vi "Test.vi"   [LabVIEW 2014]
doc: "This VI is called when test mode begins, and will automatically be terminated when it ends. You can add manual or automatic tests and invoke them from the dashboard."
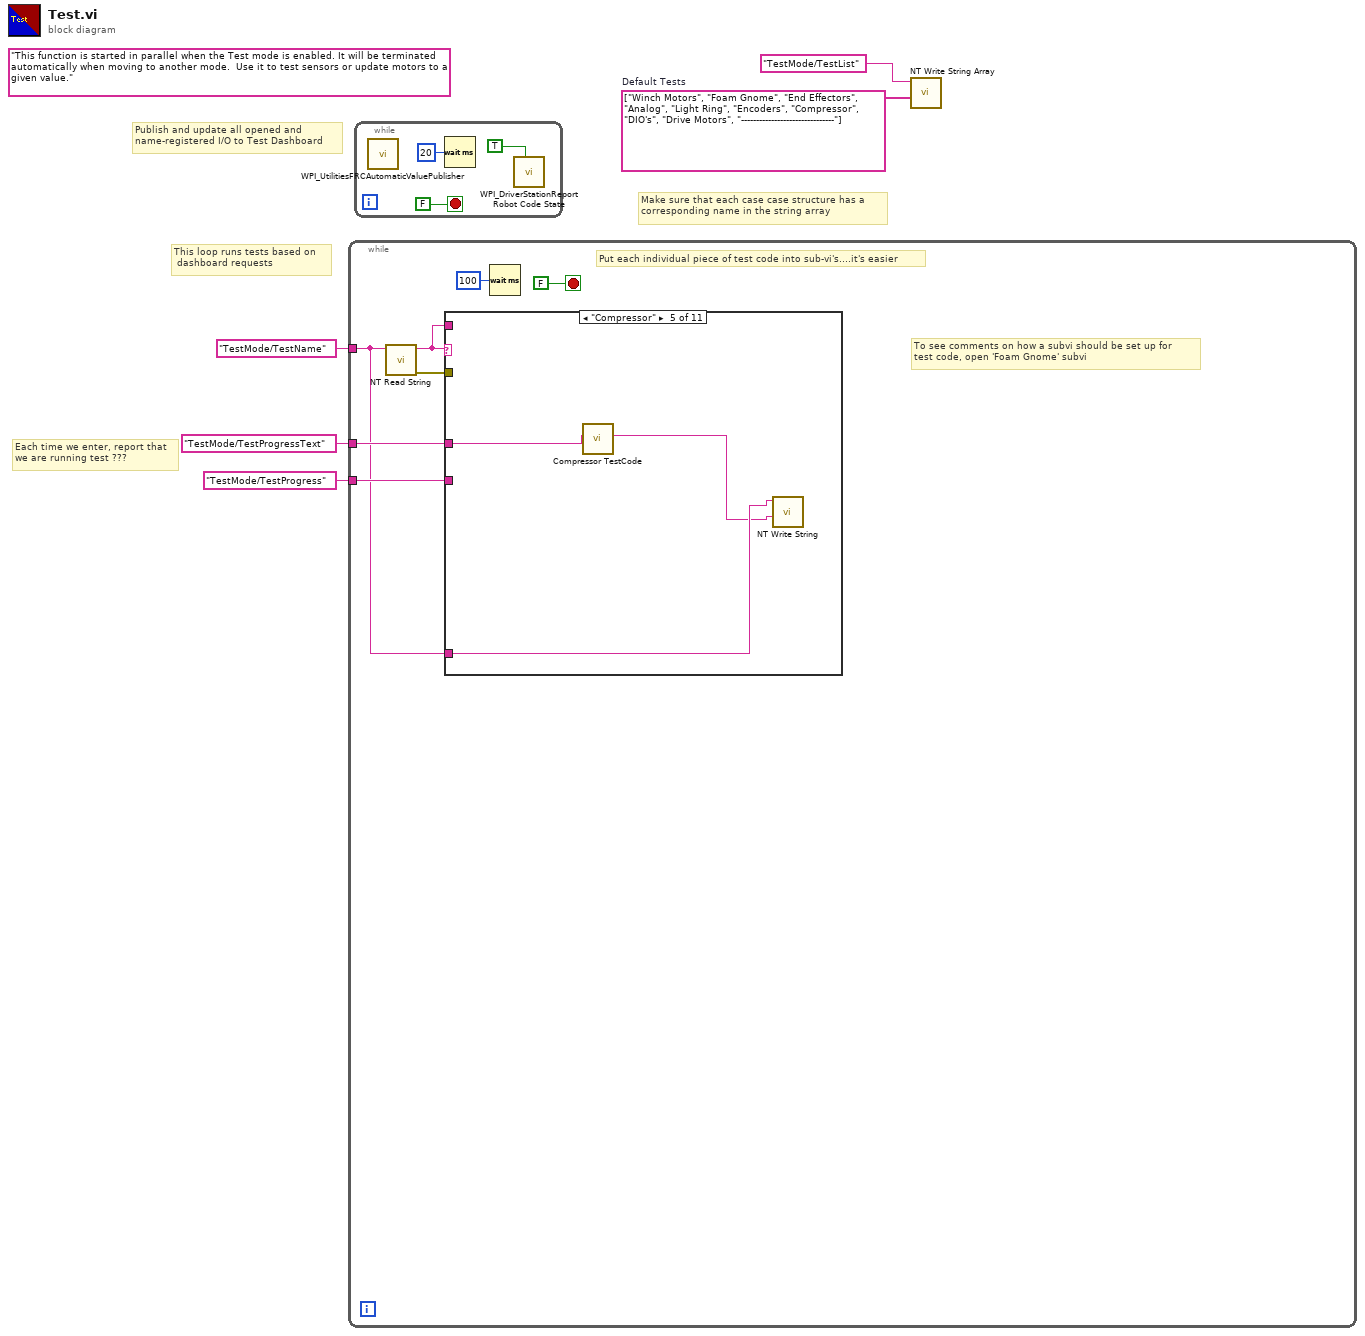
[diagram p0: block diagram]
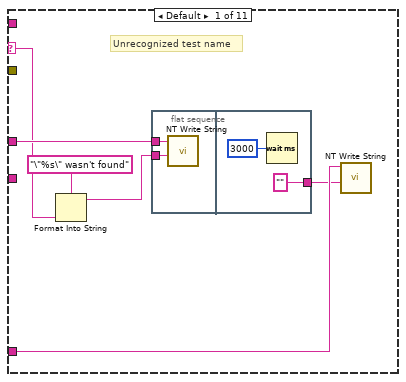
[diagram p2: hidden frame]
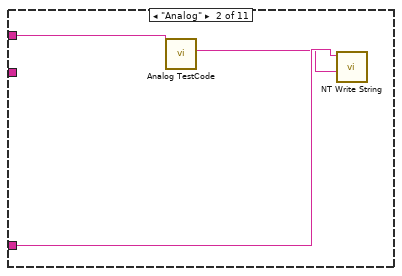
[diagram p3: hidden frame]
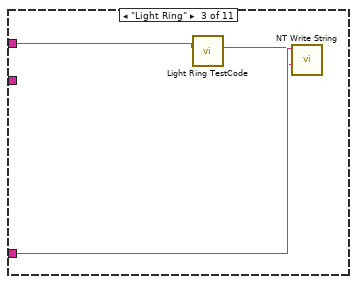
[diagram p4: hidden frame]
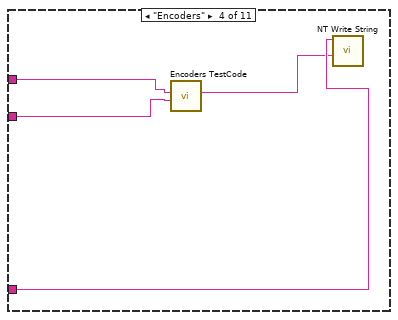
[diagram p5: hidden frame]
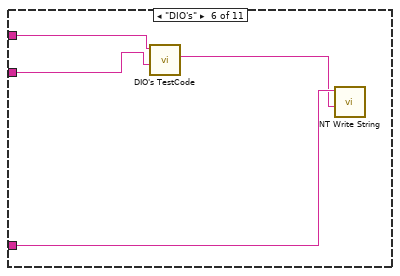
[diagram p6: hidden frame]
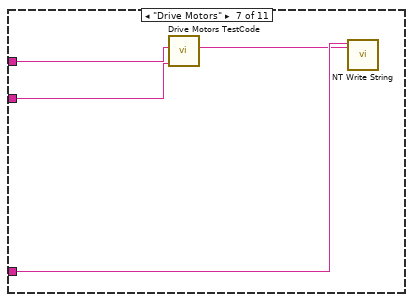
[diagram p7: hidden frame]
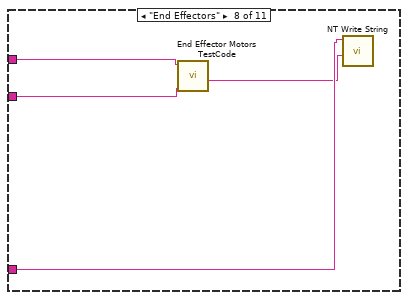
[diagram p8: hidden frame]
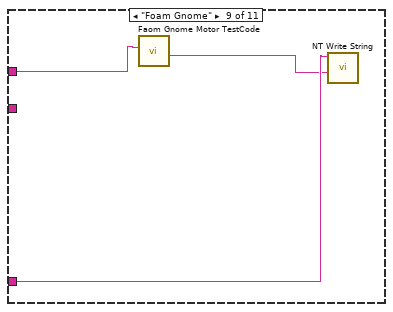
[diagram p9: hidden frame]
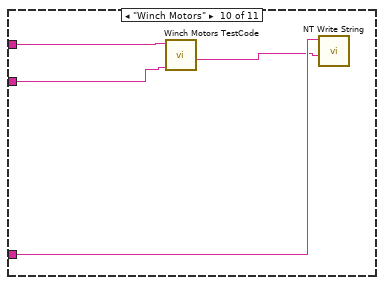
[diagram p10: hidden frame]
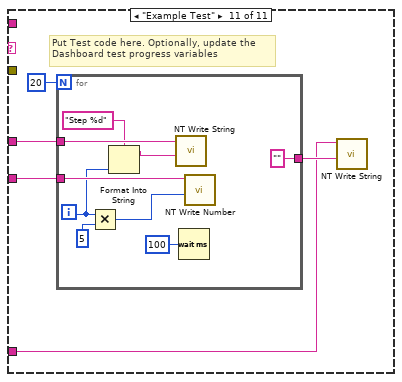
[diagram p11: hidden frame]
diagram:
  w2 = string[] ["Winch Motors", "Foam Gnome", "End Effectors", "Analog", "Light Ring", "Encoders", "Compressor", "DIO's", "Drive Motors", "-------------------------------"]  # Default Tests
  (unwired) "This function is started in parallel when the Test mode is enabled. It will be terminated automatically when moving to another mode.  Use it to test sensors or update motors to a given value."
  # "Make sure that each case case structure has a \ncorresponding name in the string array"
  # "This loop runs tests based on \n dashboard requests"
  # "Publish and update all opened and\nname-registered I/O to Test Dashboard"
  # "Each time we enter, report that\nwe are running test ???"
  n1 = while {
    tunnel: "TestMode/TestName" ("Name") -> [w7]
    tunnel: "TestMode/TestProgressText" ("Name") -> [w10]
    tunnel: "TestMode/TestProgress" ("Name") -> [w9]
    stop <- FALSE stop-if-true
    # "To see comments on how a subvi should be set up for\ntest code, open 'Foam Gnome' subvi"
    # "Put each individual piece of test code into sub-vi's....it's easier"
    n2 = call <vilib>:"NT Read String.vi"("Name"=w7) -> ("error out"=w6:errorcluster, "String"=w8:string)  [unwired: 9 in]
    n3 = case shown="\"Compressor\"" w8 {
      selector: w8 -> [w17 _ _ _ _ _ _ _ _ _ _]
      tunnel: w7 -> [w14 w25 w27 w32 w35 w39 w43 w47 w50 w54 w55]
      tunnel: w10 -> [w18 w23 w28 w31 w34 w38 w42 w46 w49 w52 w58]
      tunnel: w9 -> [_ _ _ w30 _ w37 w41 w45 _ w51 w59]
      tunnel: w8 -> [_ _ _ _ _ _ _ _ _ _ _]
      tunnel: w6 -> [_ _ _ _ _ _ _ _ _ _ _]
      frame Default {
        # "Unrecognized test name"
        n4 = Format Into String(format string="\"%s\" wasn't found" ("Name"), w17) -> (resulting string=w16:string)  [unwired: 2 in, 1 out]
        n5 = flat-sequence {
          tunnel: w18 -> [w19]
          tunnel: w16 -> [w20]
          tunnel: ["" ("Name")] -> w13
          frame #0 {
            n6 = call <vilib>:"NT Write String.vi"("String"=w20, "Name"=w19) -> ()  [unwired: 9 in, 1 out]
          }
          frame #1 {
            n7 = Wait (ms)(milliseconds to wait=u32 3000) -> ()  [unwired: 1 out]
          }
        }
        n8 = call <vilib>:"NT Write String.vi"("String"=w13, "Name"=w14) -> ()  [unwired: 9 in, 1 out]
      }
      frame "Analog" {
        n9 = call "Analog TestCode.vi"(10:w23) -> ("String"=w24:string)  [unwired: 10 in]
        n10 = call <vilib>:"NT Write String.vi"("String"=w24, "Name"=w25) -> ()  [unwired: 9 in, 1 out]
      }
      frame "Light Ring" {
        n11 = call "Light Ring TestCode.vi"("Step Text"=w28) -> ("Light Ring Output"=w26:string)  [unwired: 10 in]
        n12 = call <vilib>:"NT Write String.vi"("String"=w26, "Name"=w27) -> ()  [unwired: 9 in, 1 out]
      }
      frame "Encoders" {
        n13 = call "Encoders TestCode.vi"(1:"Step Text"=w31, 2:"Step Text"=w30) -> ("Encoders Output"=w29:string)  [unwired: 8 in]
        n14 = call <vilib>:"NT Write String.vi"("String"=w29, "Name"=w32) -> ()  [unwired: 9 in, 1 out]
      }
      frame "Compressor" {
        n15 = call "Compressor TestCode.vi"("Step Text"=w34) -> ("Compressor Output"=w33:string)  [unwired: 10 in]
        n16 = call <vilib>:"NT Write String.vi"("String"=w33, "Name"=w35) -> ()  [unwired: 9 in, 1 out]
      }
      frame "DIO's" {
        n17 = call "DIO's TestCode.vi"(9:"Step Text"=w37, 11:"Step Text"=w38) -> ("DIO Output"=w36:string)  [unwired: 9 in]
        n18 = call <vilib>:"NT Write String.vi"("String"=w36, "Name"=w39) -> ()  [unwired: 9 in, 1 out]
      }
      frame "Drive Motors" {
        n19 = call "Drive Motors TestCode.vi"(8:"Step Text"=w41, 10:"Step Text"=w42) -> ("Drive Motors Output"=w40:string)  [unwired: 9 in]
        n20 = call <vilib>:"NT Write String.vi"("String"=w40, "Name"=w43) -> ()  [unwired: 9 in, 1 out]
      }
      frame "End Effectors" {
        n21 = call "End Effector Motors TestCode.vi"(0:"Step Text"=w46, 3:"Step Text"=w45) -> ("Drive Motors Output"=w44:string)  [unwired: 7 in]
        n22 = call <vilib>:"NT Write String.vi"("String"=w44, "Name"=w47) -> ()  [unwired: 9 in, 1 out]
      }
      frame "Foam Gnome" {
        n23 = call "Faom Gnome Motor TestCode.vi"("Step Text"=w49) -> ("Foam Gnome Output"=w48:string)  [unwired: 10 in]
        n24 = call <vilib>:"NT Write String.vi"("String"=w48, "Name"=w50) -> ()  [unwired: 9 in, 1 out]
      }
      frame "Winch Motors" {
        n25 = call "Winch Motors TestCode.vi"(8:"Step Text"=w51, 11:"Step Text"=w52) -> ("Winch Motors Output"=w53:string)  [unwired: 9 in]
        n26 = call <vilib>:"NT Write String.vi"("String"=w53, "Name"=w54) -> ()  [unwired: 9 in, 1 out]
      }
      frame "Example Test" {
        # "Put Test code here. Optionally, update the\nDashboard test progress variables"
        n27 = for {
          N: 20 -> [_]
          tunnel: w59 -> [w68]
          tunnel: w58 -> [w66]
          tunnel: ["" ("String")] -> w56
          i -> [w63]
          n28 = Multiply(x=w63, y=u32 5 ("milliseconds to wait")) -> (x*y=w64:u32)
          n29 = Format Into String(format string="Step %d", w63) -> (resulting string=w61:string)  [unwired: 2 in, 1 out]
          n30 = call <vilib>:"NT Write String.vi"("String"=w61, "Name"=w66) -> ()  [unwired: 9 in, 1 out]
          n31 = Wait (ms)(milliseconds to wait=u32 100) -> ()  [unwired: 1 out]
          n32 = call <vilib>:"NT Write Number.vi"("Numeric"=w64, "Name"=w68) -> ()  [unwired: 9 in, 1 out]
        }
        n33 = call <vilib>:"NT Write String.vi"("String"=w56, "Name"=w55) -> ()  [unwired: 9 in, 1 out]
      }
    }
    n34 = Wait (ms)(milliseconds to wait=u32 100) -> ()  [unwired: 1 out]
  }
  n35 = while {
    stop <- FALSE stop-if-true
    n36 = call <vilib>:"WPI_UtilitiesFRCAutomaticValuePublisher.vi"() -> ()  [unwired: 12 in]
    n37 = Wait (ms)(milliseconds to wait=u32 20) -> ()  [unwired: 1 out]
    n38 = call <vilib>:"WPI_DriverStationReport Robot Code State.vi"("Test"=TRUE ("Autonomous")) -> ()  [unwired: 10 in, 1 out]
  }
  n39 = call <vilib>:"NT Write String Array.vi"("String Array"=w2, "Name"="TestMode/TestList") -> ()  [unwired: 9 in, 1 out]
